vi "CRYData throw-away decide.vi"(9 "Maximum % processed (20%)":dbl=20.0 format="%.2f", 10 "Iteration":i32, 11 "Buffer use (%)":i32) -> (2 "Portion of data processed (%)":dbl format="%.2f", 3 "Suppress processing":bool)   [LabVIEW 2013]
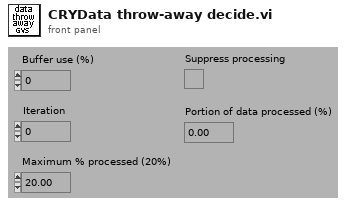
[diagram p1: front panel]
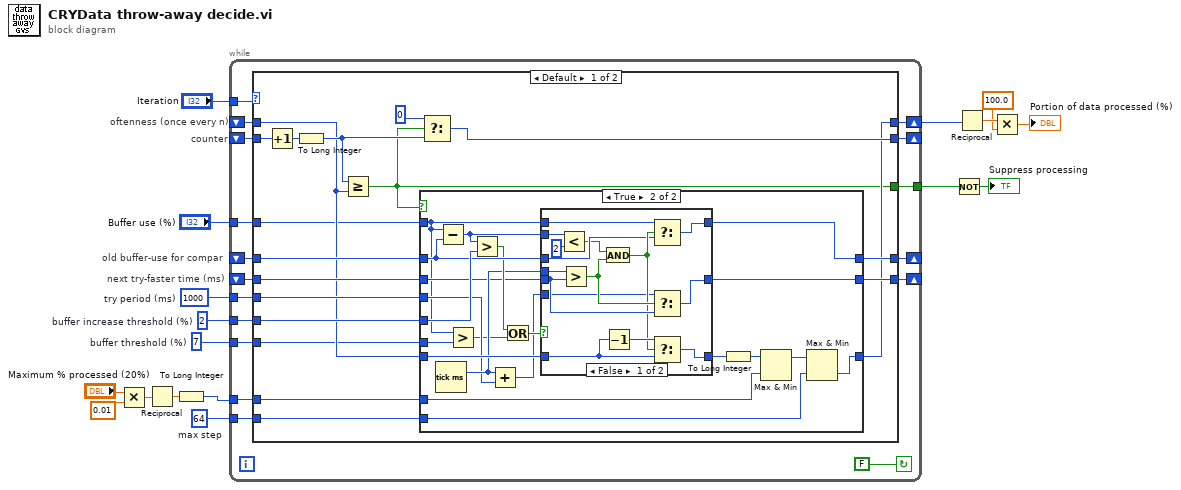
[diagram p0: block diagram]
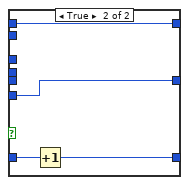
[diagram p3: hidden frame]
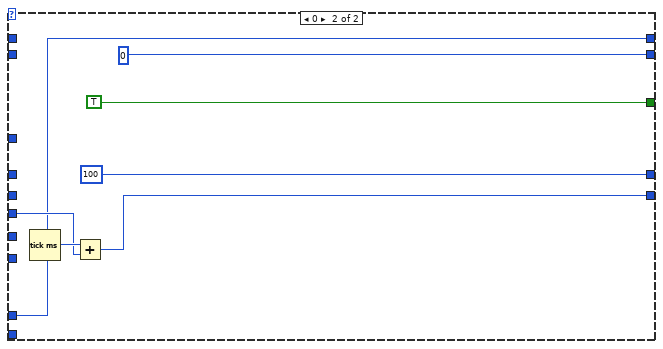
[diagram p4: hidden frame]
diagram:
  w6 = 7  # buffer threshold (%)
  w7 = 64  # max step
  w8 = 2  # buffer increase threshold (%)
  w10 = u32 1000  # try period (ms)
  # "next try-faster time (ms)"
  # "old buffer-use for compar"
  # "counter"
  # "oftenness (once every n)"
  n1 = Multiply(x="Maximum % processed (20%)", y=0.01) -> (x*y=w3:dbl)
  n2 = Reciprocal(x=w3) -> (1/x=w2:dbl)
  n3 = To Long Integer(number=w2) -> (32bit integer=w1:i32)
  n4 = while {
    tunnel: w6 -> [w19]
    tunnel: w7 -> [w20]
    tunnel: w1 -> [w21]
    tunnel: w8 -> [w23]
    tunnel: "Buffer use (%)" -> [w25]
    shift-left: _ -> [w22]
    shift-right: [w27] -> _
    tunnel: w10 -> [w28]
    shift-left: _ -> [w24]
    shift-right: [w26] -> _
    tunnel: [w29] -> w16
    shift-left: _ -> [w30]
    shift-right: [w31] -> _
    shift-left: _ -> [w32]
    shift-right: [w33] -> w14
    tunnel: "Iteration" -> [w34]
    stop <- FALSE continue-if-true
    n5 = case shown="Default" w34 {
      tunnel: [w38 w96] -> w33
      tunnel: w32 -> [w41 _]
      tunnel: [w49 0] -> w31
      tunnel: w30 -> [w52 _]
      tunnel: [w36 TRUE] -> w29
      tunnel: w28 -> [w45 w100]
      tunnel: [w43 w99] -> w27
      tunnel: [w46 100 ("Buffer use (%)")] -> w26
      tunnel: w25 -> [w37 _]
      tunnel: w24 -> [w48 _]
      tunnel: w23 -> [w47 _]
      tunnel: w22 -> [w44 _]
      tunnel: w21 -> [w40 w96]
      tunnel: w20 -> [w39 _]
      tunnel: w19 -> [w35 _]
      frame Default {
        n6 = Increment(x=w52) -> (x+1=w50:i32)
        n7 = To Long Integer(number=w50) -> (32bit integer=w42:i32)
        n8 = Greater Or Equal?(x=w42, y=w41) -> (x >= y?=w36:bool)
        n9 = case shown="True" w36 {
          tunnel: w37 -> [_ w57]
          tunnel: w48 -> [w55 w75]
          tunnel: w47 -> [_ w76]
          tunnel: [w55 w66] -> w46
          tunnel: w45 -> [_ w61]
          tunnel: w44 -> [w54 w62]
          tunnel: [w54 w74] -> w43
          tunnel: w41 -> [w53 w73]
          tunnel: [w53 w67] -> w38
          tunnel: w40 -> [_ w69]
          tunnel: w39 -> [_ w68]
          tunnel: w35 -> [_ w58]
          frame False {
          }
          frame True {
            n10 = Tick Count (ms)() -> (millisecond timer value=w63:u32)
            n11 = Subtract(x=w57, y=w75) -> (x-y=w59:i32)
            n12 = Greater?(x=w57, y=w58) -> (0:w56:bool)
            n13 = Greater?(x=w59, y=w76) -> (0:w65:bool)
            n14 = Add(x=w63, y=w61) -> (x+y=w60:u32)
            n15 = Or(x=w65, y=w56) -> (x .or. y?=w64:bool)
            n16 = case shown="False" w64 {
              tunnel: w75 -> [w82 _]
              tunnel: w62 -> [w86 _]
              tunnel: [w87 w92] -> w74
              tunnel: w73 -> [w91 w95]
              tunnel: [w90 w94] -> w70
              tunnel: [w83 w93] -> w66
              tunnel: w57 -> [w85 w93]
              tunnel: w63 -> [w81 _]
              tunnel: w60 -> [w80 w92]
              tunnel: w59 -> [w79 _]
              frame False {
                n17 = Less?(x=w79, y=2 ("buffer increase threshold (%)")) -> (x < y?=w77:bool)
                n18 = Greater?(x=w81, y=w86) -> (0:w88:bool)
                n19 = And(x=w77, y=w88) -> (x .and. y?=w84:bool)
                n20 = Decrement(x=w91) -> (x-1=w89:i32)
                n21 = Select(t=w85, s=w84, f=w82) -> (s? t:f=w83:i32)
                n22 = Select(t=w80, s=w88, f=w86) -> (s? t:f=w87:u32)
                n23 = Select(t=w89, s=w84, f=w91) -> (s? t:f=w90:i32)
              }
              frame True {
                n24 = Increment(x=w95) -> (x+1=w94:i32)
              }
            }
            n25 = To Long Integer(number=w70) -> (32bit integer=w72:i32)
            n26 = Max & Min(x=w72, y=w69) -> (max(x,y)=w71:i32)  [unwired: 1 out]
            n27 = Max & Min(x=w71, y=w68) -> (min(x,y)=w67:i32)  [unwired: 1 out]
          }
        }
        n28 = Select(t=0, s=w36, f=w42) -> (s? t:f=w49:i32)
      }
      frame 0 {
        n29 = Tick Count (ms)() -> (millisecond timer value=w101:u32)
        n30 = Add(x=w101, y=w100) -> (x+y=w99:u32)
      }
    }
  }
  n31 = Not(x=w16) -> (.not. x?=→"Suppress processing":bool)
  n32 = Reciprocal(x=w14) -> (1/x=w13:dbl)
  n33 = Multiply(x=w13, y=100.0) -> (x*y=→"Portion of data processed (%)":dbl)
